vi "Insight_RW_Kp.vi"(8 "error in (no error)":errorcluster, 9 "Mode (Read / Write)":enum8{"Write", "Read"}(ring), 10 "Kp":dbl=1520.0, 11 "telnet connection":T1) -> (0 "error out":errorcluster, 1 "response data":string, 2 "Kp":dbl, 3 "telnet  connection out":T1)   [LabVIEW 2011]
doc: "Insight Photonic Solutions\n\nThis VI reads or writes the Kp value used in the power-leveling routine. Kp sets the strength of the proportional correction in the power control. By definition, Kp must be negative. By experience, Kp is between -1 and -15.\n\nver 1.0 - original release"
uses:
  Telnet Session.ctl
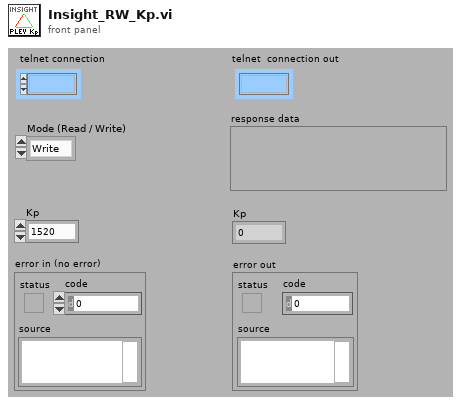
[diagram p1: front panel]
types:
  T1 = typedef "Telnet Session.ctl" = refnum<k1>
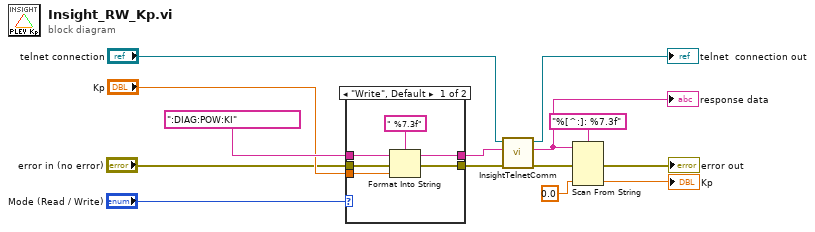
[diagram p0: block diagram]
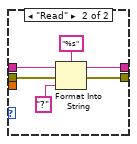
[diagram p2: hidden frame]
diagram:
  n1 = case shown="\"Write\", Default" "Mode (Read / Write)" {
    tunnel: [w20 w22] -> w8
    tunnel: "error in (no error)" -> [w19 w21]
    tunnel: ":DIAG:POW:KI" ("String") -> [w18 w24]
    tunnel: "Kp" -> [w17 _]
    tunnel: [w15 w23] -> w5
    frame "Write", Default {
      n2 = Format Into String(format string=" %7.3f", initial string=w18, error in=w19, w17) -> (resulting string=w15:string, error out=w20:errorcluster)
    }
    frame "Read" {
      n3 = Format Into String(format string="%s", initial string=w24, error in=w21, "?" ("input 1")) -> (resulting string=w23:string, error out=w22:errorcluster)
    }
  }
  n4 = call "InsightTelnetComm.vi"("error in"=w8, "write buffer (\"\")"=w5, "telnet connection"="telnet connection") -> ("error out"=w7:errorcluster, "response data"=w6:string, "telnet  connection out"=→"telnet  connection out":T1)  [unwired: 4 in]
  "response data" <- w6
  n5 = Scan From String(format string="%[^:]: %7.3f", input string=w6, error in=w7, default 2=0.0 ("default value 1")) -> (error out=→"error out":errorcluster, output 2=→"Kp":dbl)  [unwired: 3 in, 2 out]
